vi "which button.vi"(0 "state":T1) -> (1 "index of element":i32)   [LabVIEW 2010]
uses:
  Calibrator state.ctl
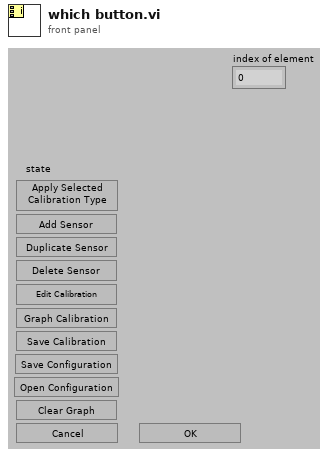
[diagram p1: front panel]
types:
  T1 = typedef "Calibrator state.ctl" = cluster{"OK":bool, "update calibration":bool, "Add Sensor":bool, "Duplicate Sensor":bool, "Delete Sensor":bool, "Delete Sensor 2":bool, "Graph calibration":bool, "Save calibration":bool, "Save Configuration":bool, "Open Configuration":bool, "Clear Graph":bool, "Cancel":bool}
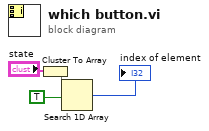
[diagram p0: block diagram]
diagram:
  n1 = Cluster To Array(cluster="state") -> (array=w2:bool[])
  n2 = Search 1D Array(1D array=w2, element=TRUE) -> (index of element=→"index of element":i32)  [unwired: 1 in]
